vi "FDG.vi"(0 "System no.":i32=1 min=1 step=1, 1 "Board":i32=1 min=1 max=5 step=1, 2 "Routinename":string, 3 "Axis settings":cluster{"Scan axis":string, "Step axis":string}, 4 "Amplitude settings":T5={"Min amplitude"=0.4, "Set min. amplitude?"=FALSE, "Max amplitude"=0.8, "Set max. amplitude?"=FALSE} {"Max amplitude" format="%.4f"; "Min amplitude" format="%.4f"}, 5 "error in":errorcluster, 6 "Minimum Level":dbl=0.1 format="%.3f", 7 "Frequency settings":cluster{"Set frequency?":bool, "Frequency":dbl}={"Set frequency?"=FALSE, "Frequency"=10.0} {"Frequency" format="%.3f"}, 8 "Velocity settings":T4={"Set max. velocity?"=FALSE, "Max velocity"=4.0} {"Max velocity" format="%.4f"}, 9 "Speed offset settings":T1={"Set speed offset?"=FALSE, "Speed offset"=0.05} {"Speed offset" format="%.4f"}, 10 "Speed factor settings":T3={"Set speed factor?"=FALSE, "Speed factor"=0.25} {"Speed factor" format="%.4f"}, 11 "Max. direction changes settings":T2={"Set max. dir. changes?"=FALSE, "Max. dir. changes"=10}) -> (19 "error out":errorcluster)   [LabVIEW 2020]
doc: "Defines a fast alignment gradient search routine. Use FRS to start the routine and FRR? to read out the results of the routine. \n\nC-887, E-712:"
panel:
  # "Defines a fast alignment gradient search procedure. Use FRS to start the procedure\nand FRR? to read out the results of the procedure."
  # "If Yes:"
  # "If Yes:"
  # "If Yes:"
  # "If Yes:"
  # "If Yes:"
  # "If Yes:"
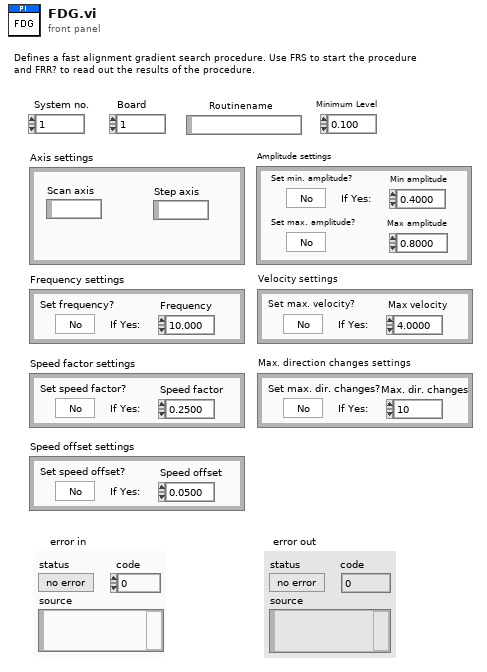
[diagram p1: front panel]
types:
  T1 = cluster{"Set speed offset?":bool, "Speed offset":dbl}
  T2 = cluster{"Set max. dir. changes?":bool, "Max. dir. changes":i32}
  T3 = cluster{"Set speed factor?":bool, "Speed factor":dbl}
  T4 = cluster{"Set max. velocity?":bool, "Max velocity":dbl}
  T5 = cluster{"Min amplitude":dbl, "Set min. amplitude?":bool, "Max amplitude":dbl, "Set max. amplitude?":bool}
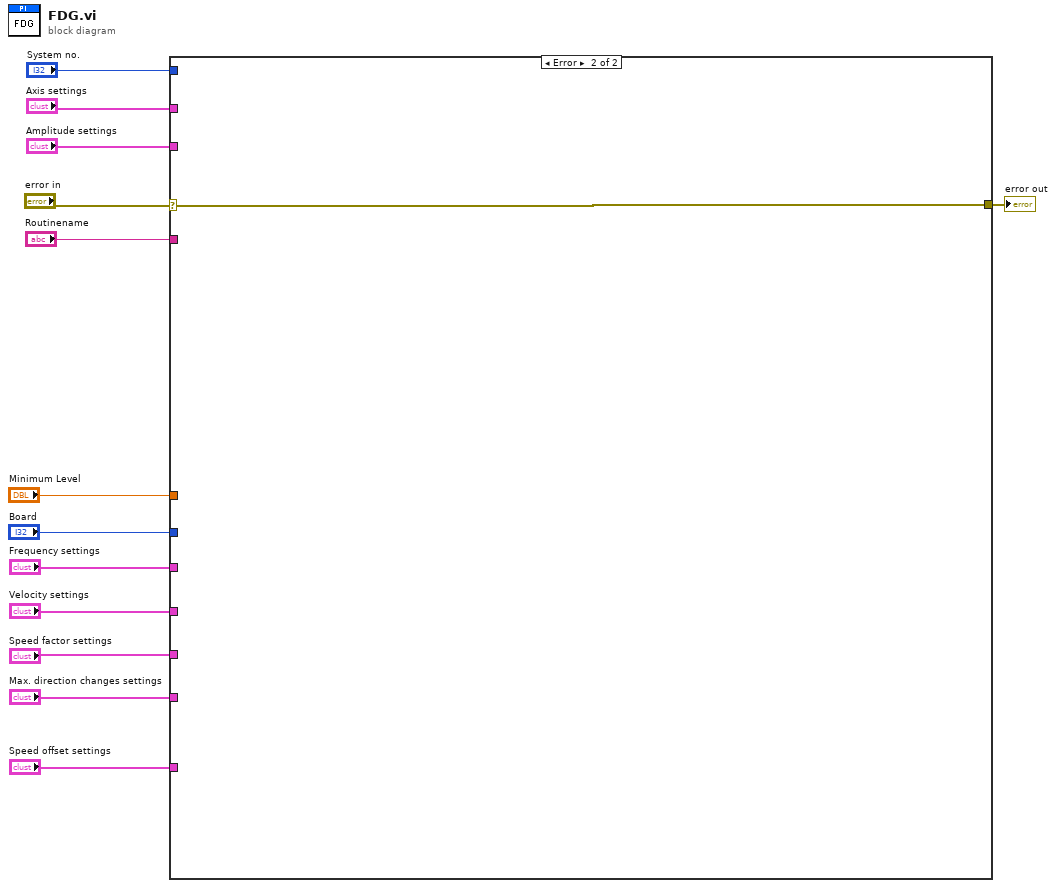
[diagram p0: block diagram]
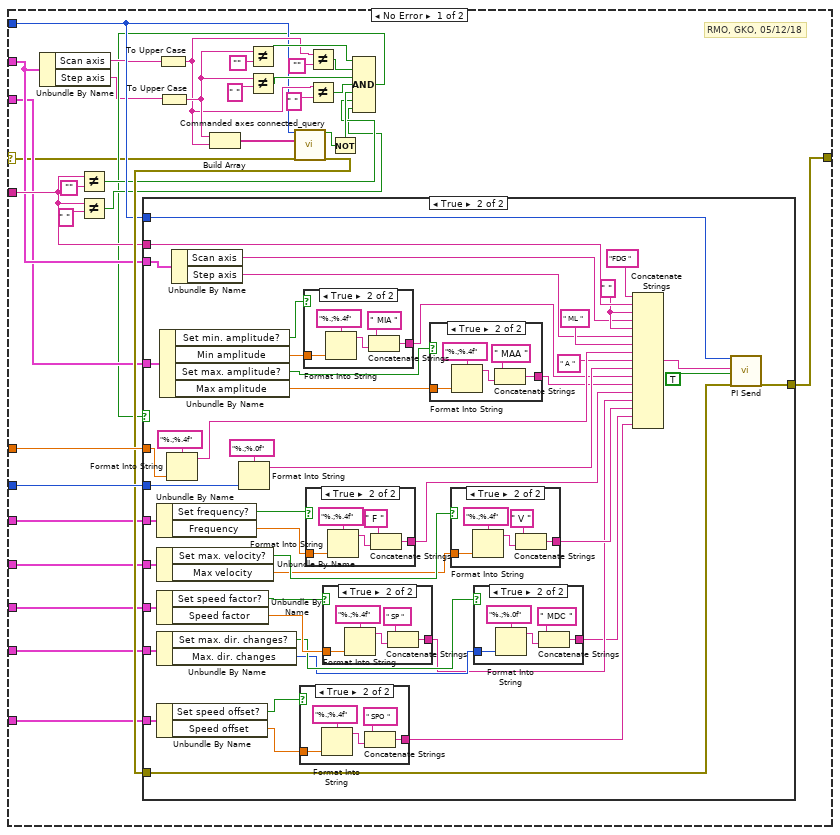
[diagram p2: hidden frame]
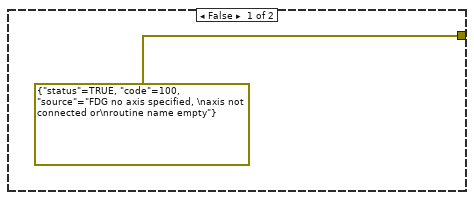
[diagram p3: hidden frame]
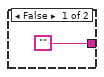
[diagram p4: hidden frame]
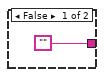
[diagram p5: hidden frame]
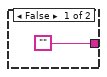
[diagram p6: hidden frame]
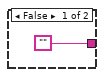
[diagram p7: hidden frame]
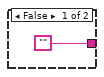
[diagram p8: hidden frame]
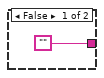
[diagram p9: hidden frame]
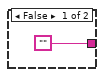
[diagram p10: hidden frame]
diagram:
  n1 = case shown="Error" "error in" {
    selector: "error in" -> [w14 w137]
    tunnel: "System no." -> [w30 _]
    tunnel: [w40 w137] -> w12
    tunnel: "Amplitude settings" -> [w22 _]
    tunnel: "Board" -> [w43 _]
    tunnel: "Velocity settings" -> [w20 _]
    tunnel: "Speed factor settings" -> [w19 _]
    tunnel: "Minimum Level" -> [w42 _]
    tunnel: "Axis settings" -> [w23 _]
    tunnel: "Routinename" -> [w24 _]
    tunnel: "Frequency settings" -> [w21 _]
    tunnel: "Max. direction changes settings" -> [w18 _]
    tunnel: "Speed offset settings" -> [w17 _]
    frame No Error {
      # "RMO, GKO, 05/12/18"
      n2 = Unbundle By Name(w23) -> ("Scan axis"=w29:string, "Step axis"=w15:string)
      n3 = Not Equal?(x=w24, y="") -> (x != y?=w26:bool)
      n4 = Not Equal?(x=w24, y=" ") -> (x != y?=w25:bool)
      n5 = To Upper Case(1:w29) -> (0:w31:string)
      n6 = To Upper Case(1:w15) -> (0:w32:string)
      n7 = Build Array(w32, w31) -> (w44:string[])
      n8 = Not Equal?(x=w32, y="") -> (x != y?=w45:bool)
      n9 = Not Equal?(x=w32, y=" ") -> (x != y?=w35:bool)
      n10 = call "Commanded axes connected_query.vi"("System no."=w30, "Commanded axes"=w44, "error in"=w14) -> ("Controller error"=w39:bool, "error out"=w41:errorcluster)  [unwired: 15 out]
      n11 = Not Equal?(x=w31, y="") -> (x != y?=w34:bool)
      n12 = Not Equal?(x=w31, y=" ") -> (x != y?=w33:bool)
      n13 = Not(x=w39) -> (.not. x?=w38:bool)
      n14 = Compound Arithmetic op=AND(w45, w34, w35, w33, w38, w26, w25) -> (w16:bool)
      n15 = case shown="True" w16 {
        tunnel: w43 -> [_ w88]
        tunnel: w42 -> [_ w84]
        tunnel: w41 -> [_ w94]
        tunnel: w30 -> [_ w90]
        tunnel: [errorcluster {"status"=TRUE, "code"=100, "source"="FDG no axis specified, \naxis not connected or\nroutine name empty"} ("error out") w49] -> w40
        tunnel: w24 -> [_ w86]
        tunnel: w23 -> [_ w53]
        tunnel: w22 -> [_ w54]
        tunnel: w21 -> [_ w83]
        tunnel: w20 -> [_ w79]
        tunnel: w19 -> [_ w74]
        tunnel: w18 -> [_ w65]
        tunnel: w17 -> [_ w58]
        frame False {
        }
        frame True {
          w85 = " "
          n16 = Unbundle By Name(w83) -> ("Set frequency?"=w82:bool, "Frequency"=w77:dbl)
          n17 = Unbundle By Name(w79) -> ("Set max. velocity?"=w80:bool, "Max velocity"=w76:dbl)
          n18 = Unbundle By Name(w74) -> ("Set speed factor?"=w73:bool, "Speed factor"=w72:dbl)
          n19 = Unbundle By Name(w65) -> ("Set max. dir. changes?"=w64:bool, "Max. dir. changes"=w63:i32)
          n20 = Unbundle By Name(w58) -> ("Set speed offset?"=w57:bool, "Speed offset"=w56:dbl)
          n21 = Unbundle By Name(w54) -> ("Set min. amplitude?"=w78:bool, "Min amplitude"=w75:dbl, "Set max. amplitude?"=w67:bool, "Max amplitude"=w66:dbl)
          n22 = Format Into String(format string="%.;%.4f" ("Format String"), w84) -> (resulting string=w70:string)  [unwired: 2 in, 1 out]
          n23 = Unbundle By Name(w53) -> ("Scan axis"=w52:string, "Step axis"=w51:string)
          n24 = Format Into String(format string="%.;%.0f" ("Format String"), w88) -> (resulting string=w68:string)  [unwired: 2 in, 1 out]
          n25 = case shown="True" w57 {
            tunnel: ["" w97] -> w55
            tunnel: w56 -> [_ w96]
            frame False {
            }
            frame True {
              n26 = Format Into String(format string="%.;%.4f" ("Format String"), w96) -> (resulting string=w98:string)  [unwired: 2 in, 1 out]
              n27 = Concatenate Strings(" SPO ", w98) -> (w97:string)
            }
          }
          n28 = case shown="True" w78 {
            tunnel: w75 -> [_ w120]
            tunnel: ["" w121] -> w50
            frame False {
            }
            frame True {
              n29 = Format Into String(format string="%.;%.4f" ("Format String"), w120) -> (resulting string=w122:string)  [unwired: 2 in, 1 out]
              n30 = Concatenate Strings(" MIA ", w122) -> (w121:string)
            }
          }
          n31 = case shown="True" w82 {
            tunnel: ["" w133] -> w81
            tunnel: w77 -> [_ w132]
            frame False {
            }
            frame True {
              n32 = Format Into String(format string="%.;%.4f" ("Format String"), w132) -> (resulting string=w134:string)  [unwired: 2 in, 1 out]
              n33 = Concatenate Strings(" F ", w134) -> (w133:string)
            }
          }
          n34 = case shown="True" w73 {
            tunnel: ["" w115] -> w60
            tunnel: w72 -> [_ w114]
            frame False {
            }
            frame True {
              n35 = Format Into String(format string="%.;%.4f" ("Format String"), w114) -> (resulting string=w116:string)  [unwired: 2 in, 1 out]
              n36 = Concatenate Strings(" SP ", w116) -> (w115:string)
            }
          }
          n37 = case shown="True" w67 {
            tunnel: ["" w109] -> w62
            tunnel: w66 -> [_ w108]
            frame False {
            }
            frame True {
              n38 = Format Into String(format string="%.;%.4f" ("Format String"), w108) -> (resulting string=w110:string)  [unwired: 2 in, 1 out]
              n39 = Concatenate Strings(" MAA ", w110) -> (w109:string)
            }
          }
          n40 = case shown="True" w80 {
            tunnel: ["" w127] -> w61
            tunnel: w76 -> [_ w126]
            frame False {
            }
            frame True {
              n41 = Format Into String(format string="%.;%.4f" ("Format String"), w126) -> (resulting string=w128:string)  [unwired: 2 in, 1 out]
              n42 = Concatenate Strings(" V ", w128) -> (w127:string)
            }
          }
          n43 = case shown="True" w64 {
            tunnel: ["" w103] -> w59
            tunnel: w63 -> [_ w102]
            frame False {
            }
            frame True {
              n44 = Format Into String(format string="%.;%.0f" ("Format String"), w102) -> (resulting string=w104:string)  [unwired: 2 in, 1 out]
              n45 = Concatenate Strings(" MDC ", w104) -> (w103:string)
            }
          }
          n46 = Concatenate Strings("FDG ", w86, w85, w52, w85, w51, " ML ", w70, " A ", w68, w50, w62, w81, w60, w61, w59, w55) -> (w87:string)
          n47 = call "PI Send.vi"("System no."=w90, "String to send"=w87, "Attach termination char.?"=TRUE ("Attach Linefeed?"), "error in"=w94) -> ("error out"=w49:errorcluster)  [unwired: 2 in, 13 out]
        }
      }
    }
    frame Error {
    }
  }
  "error out" <- w12
